vi "Check.vi"(8 "error in (no error)":errorcluster, 10 "StartLotTraveler In":T1, 11 "EpiWrapper in":refnum<class "EpiWrapper.lvclass">) -> (0 "error out":errorcluster, 2 "StartLotTraveler Out":T1, 3 "EpiWrapper out":refnum<class "EpiWrapper.lvclass">)   [LabVIEW 2012, in "EpiWrapper.lvclass"]
uses:
  EpiWrapper.lvclass
  LotData.lvclass
  Controls/StartLotTraveler.ctl
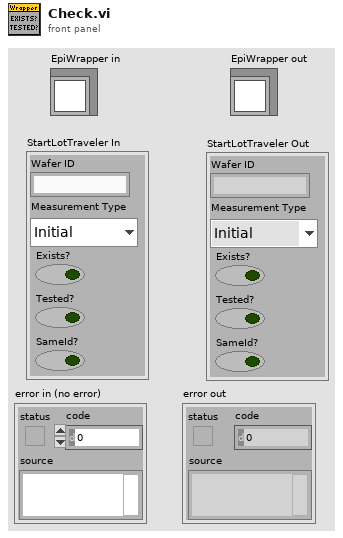
[diagram p1: front panel]
types:
  T1 = typedef "StartLotTraveler.ctl" = cluster{"Wafer ID":string, "Measurement Type":enum16{"Initial", "Final"}, "Exists?":bool, "Tested?":bool, "SameId?":bool}
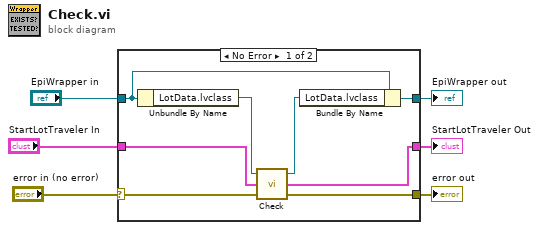
[diagram p0: block diagram]
diagram:
  n1 = case shown="No Error" "error in (no error)" {
    selector: "error in (no error)" -> [w13 w17]
    tunnel: [w9 w17] -> w5
    tunnel: [w10 w16] -> w3
    tunnel: "EpiWrapper in" -> [w12 w16]
    tunnel: "StartLotTraveler In" -> [w8 w15]
    tunnel: [w7 w15] -> w1
    frame No Error {
      n2 = Unbundle By Name(w12) -> ("LotData.lvclass"=w14:refnum<class "LotData.lvclass">)
      n3 = call "Check.vi"("error in (no error)"=w13, "StartLotTraveler In"=w8, "LotData in"=w14) -> ("error out"=w9:errorcluster, "StartLotTraveler Out"=w7:T1, "LotData out"=w11:refnum<class "LotData.lvclass">)
      n4 = Bundle By Name(cluster=w12, "LotData.lvclass"=w11) -> (w10:refnum<class "EpiWrapper.lvclass">)
    }
    frame Error {
    }
  }
  "error out" <- w5
  "EpiWrapper out" <- w3
  "StartLotTraveler Out" <- w1
